vi "verify acquisition progress.vi"(8 "error in (no error)":errorcluster, 11 "SPARC4_Channel in":refnum<class "ECHARPE_Channel.lvclass">) -> (0 "error out":errorcluster, 2 "acq in progress":cluster{"frames":bool, "cycles":bool}, 3 "SPARC4_Channel out":refnum<class "ECHARPE_Channel.lvclass">)   [LabVIEW 2018, in "ECHARPE_Channel.lvclass"]
uses:
  ECHARPE_Channel.lvclass
  Sim_CCD/Sim_CCD.lvclass
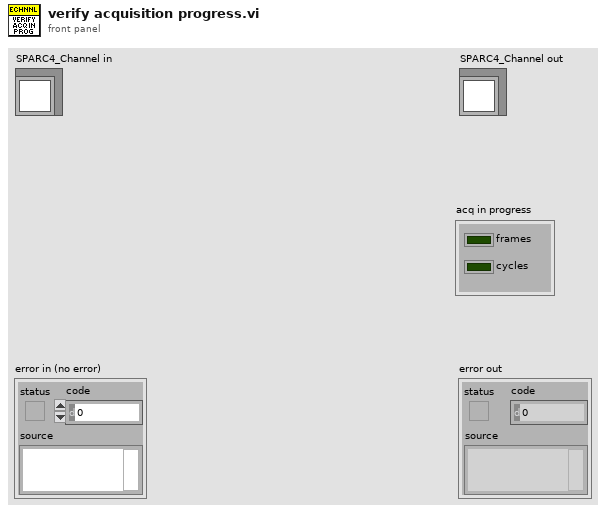
[diagram p1: front panel]
types:
  T1 = cluster{"CYCLES_DONE":u16, "LAST_IMAGE_NAME":string, "USED_DISK_SPACE":u16, "IMAGE_INDEX":u32, "acquisition error":bool}
  T2 = cluster{"State Machine.lvclass":refnum<class "State Machine.lvclass">, "RxTx.lvclass":refnum<class "RxTx.lvclass">, "Save_Header_RxTx.lvclass":refnum<class "RxTx.lvclass">, "Status SM.lvclass":refnum<class "State Machine.lvclass">, "Status RxTx.lvclass":refnum<class "RxTx.lvclass">, "servers array":refnum<class "Server.lvclass">[], "Events log file.lvclass":refnum<class "Log File.lvclass">, "Errors log file.lvclass":refnum<class "Log File.lvclass">, "Keywords log file.lvclass":refnum<class "Log File.lvclass">, "Sim_CCD.lvclass":refnum<class "Sim_CCD.lvclass">}
  T3 = cluster{"EXPTIME":dbl, "#FRAMES":u32, "COOLER_POWER_STATUS":u16, "TEMP":i32}
  T4 = cluster{"FRAMES_DONE":u16, "CCD_STATUS":string, "CURRENT_TEMPERATURE":i16, "TEMPERATURE_STATUS":string, "FRAME_EXPOSURE_TIME":dbl, "SERIAL_NUMBER":u16, "ACQUIRING":bool, "POWER":bool, "ACS MODE":bool}
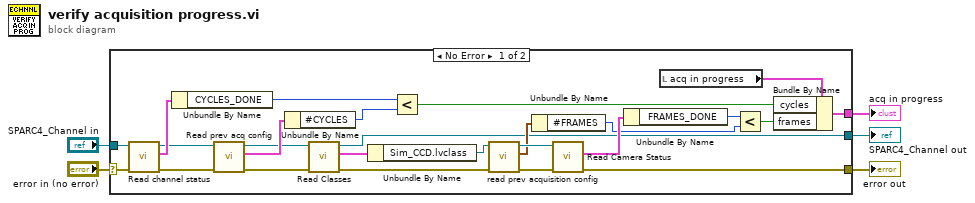
[diagram p0: block diagram]
diagram:
  n1 = case shown="No Error" "error in (no error)" {
    selector: "error in (no error)" -> [w6 w32]
    tunnel: [w20 w32] -> w4
    tunnel: [w19 w31] -> w2
    tunnel: "SPARC4_Channel in" -> [w7 w31]
    tunnel: [w15 _] -> w1
    frame No Error {
      n2 = call-dynamic "Read channel status.vi"("error in (no error)"=w6, "Channel in"=w7) -> ("error out"=w9:errorcluster, "channel status"=w10:T1, "Channel out"=w8:refnum<class "ECHARPE_Channel.lvclass">)  [unwired: 7 in]
      n3 = Unbundle By Name(w10) -> ("CYCLES_DONE"=w18:u16)
      n4 = call-dynamic "Read prev acq config.vi"("error in (no error)"=w9, "Channel in"=w8) -> ("error out"=w29:errorcluster, "prev acq config"=w30:cluster{"suffix":string, "#CYCLES":u32}, "Channel out"=w28:refnum<class "ECHARPE_Channel.lvclass">)  [unwired: 7 in]
      n5 = Unbundle By Name(w30) -> ("#CYCLES"=w17:u32)
      n6 = call-dynamic "Read Classes.vi"("error in (no error)"=w29, "Channel in"=w28) -> ("error out"=w23:errorcluster, "Classes"=w27:T2, "Channel out"=w19:refnum<class "ECHARPE_Channel.lvclass">)  [unwired: 7 in]
      n7 = Unbundle By Name(w27) -> ("Sim_CCD.lvclass"=w25:refnum<class "Sim_CCD.lvclass">)
      n8 = Less?(x=w18, y=w17) -> (x < y?=w14:bool)
      n9 = call "read prev acquisition config.vi"("error in (no error)"=w23, "Simulated_CCD_Camera in"=w25) -> ("error out"=w22:errorcluster, "prev acquisition configuration"=w21:T3, "Simulated_CCD_Camera out"=w24:refnum<class "Sim_CCD.lvclass">)  [unwired: 7 in]
      n10 = Unbundle By Name(w21) -> ("#FRAMES"=w11:u32)
      n11 = call "Read Camera Status.vi"("error in (no error)"=w22, "CCDCamera in"=w24) -> ("error out"=w20:errorcluster, "camera status"=w26:T4)  [unwired: 7 in, 1 out]
      n12 = Unbundle By Name(w26) -> ("FRAMES_DONE"=w12:u16)
      n13 = local read "acq in progress"() -> (w16:cluster{"frames":bool, "cycles":bool})
      n14 = Less?(x=w12, y=w11) -> (x < y?=w13:bool)
      n15 = Bundle By Name(cluster=w16, "cycles"=w14, "frames"=w13) -> (w15:cluster{"frames":bool, "cycles":bool})
    }
    frame Error {
    }
  }
  "error out" <- w4
  "SPARC4_Channel out" <- w2
  "acq in progress" <- w1
